vi "Periodic Tasks.vi"(8 "error in":errorcluster) -> ()   [LabVIEW 2014]
doc: "This VI runs in parallel to other tasks. It can contain as many user-defined periodic loops as you need. These can carry out PID or other sorts of timed response."
uses:
  <vilib>/Rock Robotics/WPI/Joystick/WPI_JoystickGetSetRefNum.vi
  <vilib>/Rock Robotics/WPI/RobotDrive/WPI_RobotDriveGetSetRefNum.vi
  Robot Global Data.vi
  <vilib>/addons/control/pid/pid.llb/PID (DBL).vi
  <vilib>/addons/control/pid/NI_PID_pid.lvlib
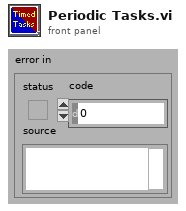
[diagram p1: front panel]
types:
  T1 = typedef "WPI_AnalogChannelDevRef.ctl" = cluster{"DevStatus":errorcluster, "Controller":T2, "Analog Channel":T3}
  T2 = typedef "FPGA_TypedefAnalogModule.ctl" = enum16{"Controller 1"}
  T3 = typedef "FPGA_AIChannel.ctl" = enum8{"AI 0", "AI 1", "AI 2", "AI 3", "AI MXP 0", "AI MXP 1", "AI MXP 2", "AI MXP 3", "Invalid"}
  T4 = typedef "WPI_MotorControlDeviceRef.ctl" = cluster{"DeviceStatus":errorcluster, "Type":T5, "PWM":cluster{"Controller":T6, "PWM Channel":T7, "DeadBand":T8}, "CAN":cluster{"Device Number":u8, "Control Mode":T9, "Semaphore":T10, "Max Vout":dbl, "TalonSRX Control Mode":T11}, "Invert":bool, "TransformRef":T12, "InvTransformRef":T12}
  T5 = typedef "WPI_MotorControlType.ctl" = enum16{"PWM", "CAN", "CANTalonSRX"}
  T6 = typedef "FPGA_TypedefDigitalModule.ctl" = enum16{"Controller 1"}
  T7 = typedef "FPGA_DIOPWMChannel.ctl" = enum8{"PWM 0", "PWM 1", "PWM 2", "PWM 3", "PWM 4", "PWM 5", "PWM 6", "PWM 7", "PWM 8", "PWM 9", "PWM MXP 0", "PWM MXP 1", "PWM MXP 2", "PWM MXP 3", "PWM MXP 4", "PWM MXP 5", "PWM MXP 6", "PWM MXP 7", "PWM MXP 8", "PWM MXP 9", "Invalid"}
  T8 = typedef "WPI_PWMDeadband.ctl" = cluster{"Name":string, "maxPositivePwm":i32, "minPositivePwm":i32, "centerPwm":i32, "maxNegativePwm":i32, "minNegativePwm":i32, "angularRange":u16}
  T9 = typedef "WPI_CANJaguar_ControlMode.ctl" = enum8{"Percent VBus", "Current", "Speed", "Position", "Voltage"}
  T10 = typedef "Semaphore RefNum" = refnum<k1>
  T11 = typedef "WPI_CANTalonSRX_APIControlMode.ctl" = enum8{"Percent VBus", "Speed", "Position", "Slave", "Unchanged / Invalid"}
  T12 = typedef "WPI_PWMTransform_ConPane.ctl" = refnum<vi>
  T13 = cluster{"proportional gain (Kc)":dbl, "integral time (Ti, min)":dbl, "derivative time (Td, min)":dbl}
  T14 = typedef "WPI_JoystickDevRef.ctl" = cluster{"Device":T15}
  T15 = typedef "WPI_JoystickDeviceEnum.ctl" = enum16{"USB 0", "USB 1", "USB 2", "USB 3", "USB 4", "USB 5"}
  T16 = typedef "WPI_RobotDriveDevRef.ctl" = cluster{"DevStatus":errorcluster, "Motors[]":T4[], "Square Inputs":bool, "Max Output":dbl}
  T17 = cluster{"JoystickDevRef":T14, "RobotDriveDevRef":T16}
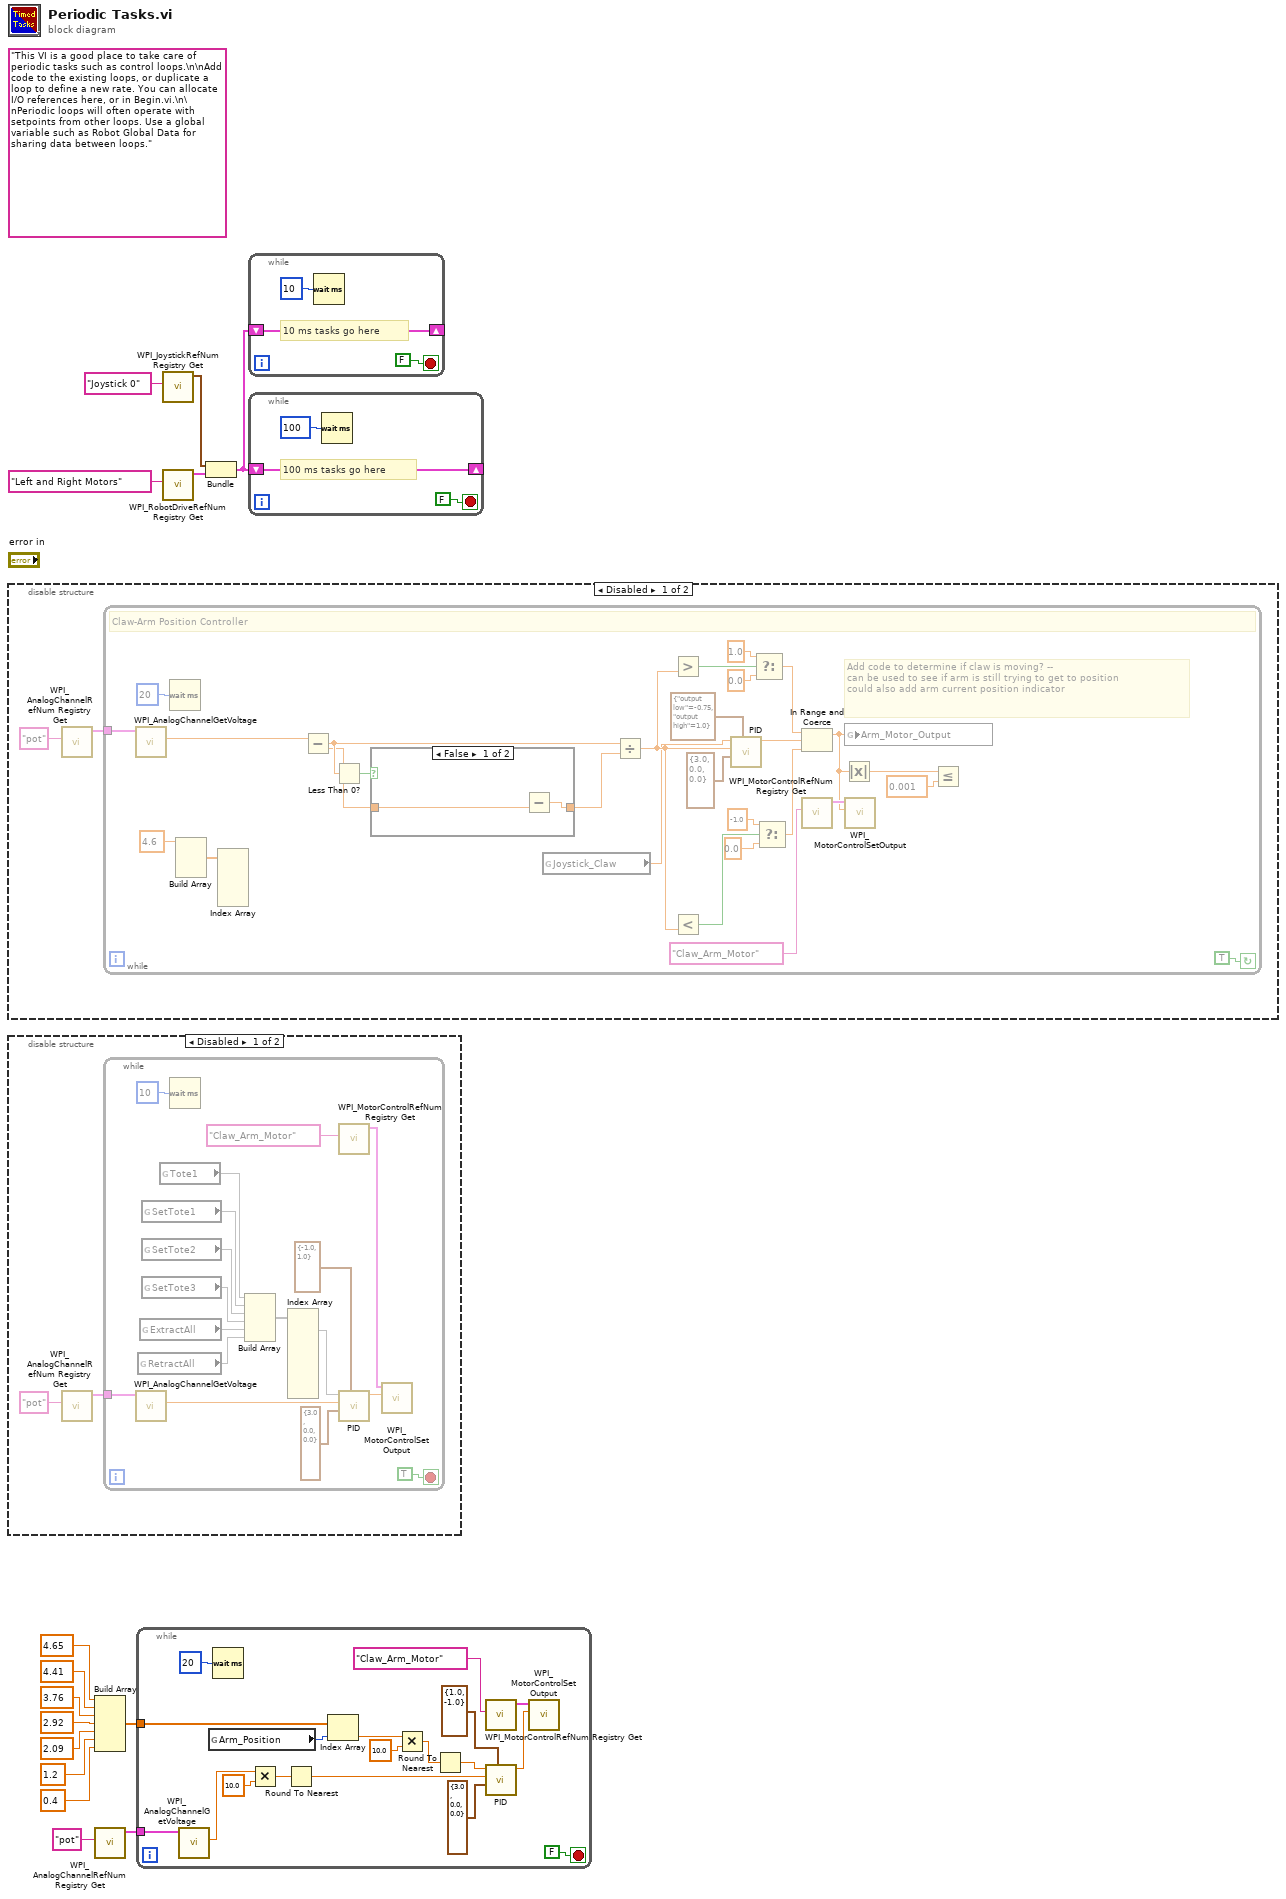
[diagram p0: block diagram]
diagram:
  (unwired) "This VI is a good place to take care of periodic tasks such as control loops.\n\nAdd code to the existing loops, or duplicate a loop to define a new rate. You can allocate I/O references here, or in Begin.vi.\n\nPeriodic loops will often operate with setpoints from other loops. Use a global variable such as Robot Global Data for sharing data between loops."
  n1 = disable-structure shown="Disabled" {
    frame Disabled {
      n2 = call <vilib>:"WPI_AnalogChannelRefNum Registry Get.vi"("refnum name"="pot") -> ("AIDeviceRef"=w16:T1)  [unwired: 1 in, 9 out]
      n3 = while {
        tunnel: w16 -> [w47]
        stop <- TRUE continue-if-true
        # "Add code to determine if claw is moving? -- \ncan be used to see if arm is still trying to get to position\ncould also add arm current position indicator"
        # "Claw-Arm Position Controller"
        n4 = call <vilib>:"WPI_AnalogChannelGetVoltage.vi"("AIDeviceRef"=w47) -> ("Voltage"=w46:dbl)  [unwired: 1 in, 9 out]
        n5 = Wait (ms)(milliseconds to wait=20) -> ()  [unwired: 1 out]
        n6 = Build Array(4.6 ("element")) -> (w18:dbl[])  [unwired: 4 in]
        n7 = Index Array(array=w18) -> ()  [unwired: 5 in, 5 out]
        n8 = global read "Robot Global Data.vi" "Joystick_Claw"() -> (w24:dbl)
        n9 = call <vilib>:"WPI_MotorControlRefNum Registry Get.vi"("refnum name"="Claw_Arm_Motor") -> ("MotorControlDevRef"=w42:T4)  [unwired: 1 in, 9 out]
        n10 = Subtract(x=w46, y=w22) -> (x-y=w39:dbl)
        n11 = Less Than 0?(x=w39) -> (x < 0?=w44:bool)
        n12 = case shown="False" w44 {
          tunnel: [w50 w51] -> w22
          tunnel: [w49 w51] -> w45
          frame False {
            n13 = Subtract(y=w50) -> (x=w48:dbl, x-y=w49:dbl)
          }
          frame True {
          }
        }
        n14 = Divide(x=w39, y=w45) -> (x/y=w25:dbl)
        n15 = Greater?(y=w25) -> (x=w20:dbl, 0:w38:bool)
        n16 = Less?(y=w25) -> (x=w21:dbl, x < y?=w35:bool)
        n17 = call-poly <vilib>:"PID.vi"("output range"=cluster{"output low":dbl, "output high":dbl} {"output low"=-0.75, "output high"=1.0}, "PID gains"=cluster{dbl, dbl, dbl} {3.0, 0.0, 0.0}, "process variable"=w25, "setpoint"=w24) -> ("output"=w32:dbl)  [unwired: 2 in, 5 out]
        n18 = Select(t=1.0, s=w38, f=0.0) -> (s? t:f=w31:dbl)
        n19 = Select(t=-1.0, s=w35, f=0.0) -> (s? t:f=w30:dbl)
        n20 = In Range and Coerce(upper limit=w31, x=w32, lower limit=w30) -> (coerced(x)=w23:dbl)  [unwired: 1 out]
        n21 = Absolute Value(x=w23) -> (abs(x)=w26:dbl)
        n22 = global write "Robot Global Data.vi" "Arm_Motor_Output"(w23) -> ()
        n23 = call <vilib>:"WPI_MotorControlSetOutput.vi"("Output"=w23, "MotorControlDevRef"=w42) -> ()  [unwired: 2 in, 8 out]
        n24 = Less Or Equal?(x=w26, y=0.001) -> ()  [unwired: 1 out]
      }
    }
    frame Enabled {
    }
  }
  n25 = disable-structure shown="Disabled" {
    frame Disabled {
      n26 = call <vilib>:"WPI_AnalogChannelRefNum Registry Get.vi"("refnum name"="pot") -> ("AIDeviceRef"=w52:T1)  [unwired: 1 in, 9 out]
      n27 = while {
        tunnel: w52 -> [w69]
        stop <- TRUE stop-if-true
        n28 = call <vilib>:"WPI_AnalogChannelGetVoltage.vi"("AIDeviceRef"=w69) -> ("Voltage"=w61:dbl)  [unwired: 1 in, 9 out]
        n29 = global read "Robot Global Data.vi" "RetractAll"() -> (w63)
        n30 = global read "Robot Global Data.vi" "ExtractAll"() -> (w55)
        n31 = global read "Robot Global Data.vi" "SetTote1"() -> (w58)
        n32 = global read "Robot Global Data.vi" "SetTote2"() -> (w57)
        n33 = global read "Robot Global Data.vi" "SetTote3"() -> (w56)
        n34 = global read "Robot Global Data.vi" "Tote1"() -> (w54)
        n35 = Wait (ms)(milliseconds to wait=u32 10) -> ()  [unwired: 1 out]
        n36 = Build Array(w54, w58, w57, w56, w55, w63) -> (w70:void[])
        n37 = Index Array(array=w70) -> (element #1=w62)  [unwired: 9 in, 8 out]
        n38 = call <vilib>:"WPI_MotorControlRefNum Registry Get.vi"("refnum name"="Claw_Arm_Motor") -> ("MotorControlDevRef"=w67:T4)  [unwired: 1 in, 9 out]
        n39 = call-poly <vilib>:"PID.vi"("output range"=cluster{"output high":dbl, "output low":dbl} {"output high"=-1.0, "output low"=1.0}, "PID gains"=T13 {"proportional gain (Kc)"=3.0, "integral time (Ti, min)"=0.0, "derivative time (Td, min)"=0.0}, "process variable"=w61, "setpoint"=w62) -> ("output"=w66:dbl)  [unwired: 2 in, 5 out]
        n40 = call <vilib>:"WPI_MotorControlSetOutput.vi"("Output"=w66, "MotorControlDevRef"=w67) -> ()  [unwired: 2 in, 8 out]
      }
    }
    frame Enabled {
    }
  }
  n41 = Build Array(4.65 ("element"), 4.41 ("element"), 3.76 ("element"), 2.92 ("element"), 2.09 ("element"), 1.2 ("element"), 0.4 ("element")) -> (w2:dbl[])
  n42 = call <vilib>:"WPI_AnalogChannelRefNum Registry Get.vi"("refnum name"="pot") -> ("AIDeviceRef"=w9:T1)  [unwired: 1 in, 9 out]
  n43 = while {
    tunnel: w9 -> [w88]
    tunnel: w2 -> [w81]
    stop <- FALSE stop-if-true
    n44 = call <vilib>:"WPI_AnalogChannelGetVoltage.vi"("AIDeviceRef"=w88) -> ("Voltage"=w75:dbl)  [unwired: 1 in, 9 out]
    n45 = global read "Robot Global Data.vi" "Arm_Position"() -> (w71:u8)
    n46 = Wait (ms)(milliseconds to wait=u32 20) -> ()  [unwired: 1 out]
    n47 = Multiply(x=w75, y=10.0) -> (x*y=w73:dbl)
    n48 = Round To Nearest(number=w73) -> (nearest integer value=w72:dbl)
    n49 = Index Array(array=w81, index=w71) -> (element=w79:dbl)
    n50 = Multiply(x=w79, y=10.0) -> (x*y=w77:dbl)
    n51 = Round To Nearest(number=w77) -> (nearest integer value=w76:dbl)
    n52 = call <vilib>:"WPI_MotorControlRefNum Registry Get.vi"("refnum name"="Claw_Arm_Motor") -> ("MotorControlDevRef"=w86:T4)  [unwired: 1 in, 9 out]
    n53 = call-poly <vilib>:"PID.vi"("output range"=cluster{"output high":dbl, "output low":dbl} {"output high"=1.0, "output low"=-1.0}, "PID gains"=T13 {"proportional gain (Kc)"=3.0, "integral time (Ti, min)"=0.0, "derivative time (Td, min)"=0.0}, "process variable"=w72, "setpoint"=w76) -> ("output"=w80:dbl)  [unwired: 2 in, 5 out]
    n54 = call <vilib>:"WPI_MotorControlSetOutput.vi"("Output"=w80, "MotorControlDevRef"=w86) -> ()  [unwired: 2 in, 8 out]
  }
  n55 = call <vilib>:"WPI_JoystickRefNum Registry Get.vi"("refnum name"="Joystick 0") -> ("JoystickDevRef"=w13:T14)  [unwired: 1 in, 9 out]
  n56 = call <vilib>:"WPI_RobotDriveRefNum Registry Get.vi"("refnum name"="Left and Right Motors") -> ("RobotDriveDevRef"=w12:T16)  [unwired: 1 in, 9 out]
  n57 = Bundle("JoystickDevRef"=w13, "RobotDriveDevRef"=w12) -> (w11:T17)  [unwired: 1 out]
  n58 = while {
    shift-right: [w89] -> _
    shift-left: w11 -> [w89]
    stop <- FALSE stop-if-true
    # "10 ms tasks go here"
    n59 = Wait (ms)(milliseconds to wait=u32 10) -> ()  [unwired: 1 out]
  }
  n60 = while {
    shift-right: [w92] -> _
    shift-left: w11 -> [w92]
    stop <- FALSE stop-if-true
    # "100 ms tasks go here"
    n61 = Wait (ms)(milliseconds to wait=u32 100) -> ()  [unwired: 1 out]
  }
